vi "get devices and variables.vi"(8 "error in (no error)":errorcluster, 11 "Device":string) -> (0 "error out":errorcluster, 1 "devicetype":string, 2 "variable":string[](array[string]), 3 "Device":string[](array[string]))   [LabVIEW 2013]
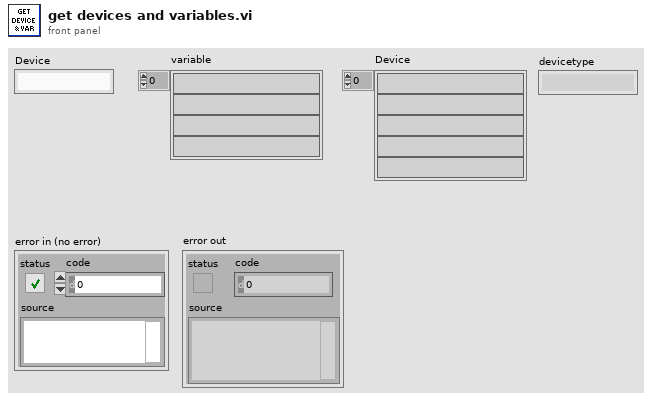
[diagram p1: front panel]
types:
  T1 = typedef "mysql_authentication.ctl" = cluster{"User":string, "Password":string, "Database":string}
  T2 = cluster{"Port":u16, "IP Address":string, "Authentication":T1}
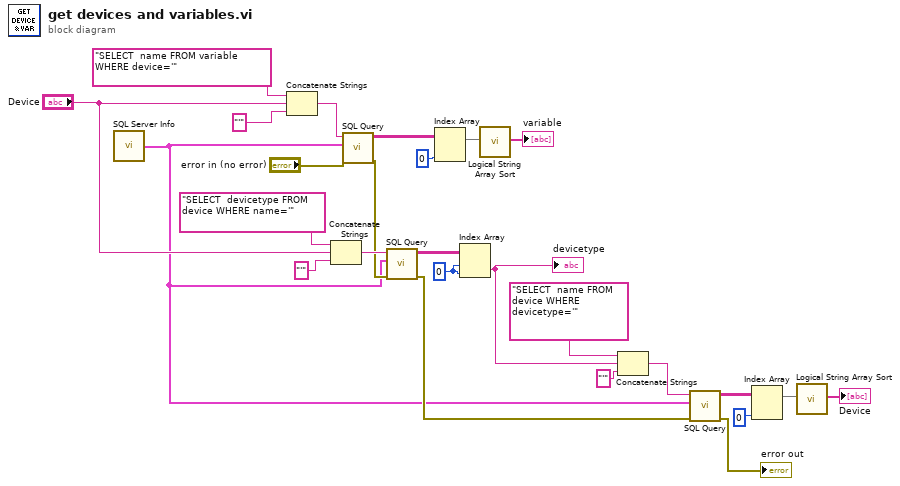
[diagram p0: block diagram]
diagram:
  w7 = 0 ("disabled index (col)")
  n1 = call "SQL Server Info.vi"() -> ("SQL Server Info"=w1:T2)
  n2 = Concatenate Strings("SELECT  name FROM variable WHERE device='" ("Query"), "Device", "'" ("string")) -> (w21:string)
  n3 = Concatenate Strings("SELECT  devicetype FROM device WHERE name='" ("Query"), "Device", "'" ("string")) -> (w8:string)
  n4 = call "SQL Query.vi"("error in (no error)"="error in (no error)", "SQL Server Info"=w1, "Query"=w21) -> ("error out"=w4:errorcluster, "data"=w26:string[][])  [unwired: 7 in]
  n5 = call "SQL Query.vi"("error in (no error)"=w4, "SQL Server Info"=w1, "Query"=w8) -> ("error out"=w3:errorcluster, "data"=w11:string[][])  [unwired: 7 in]
  n6 = Index Array(array=w26, index (col)=0 ("disabled index (col)")) -> (element=w24:string[])  [unwired: 1 in]
  n7 = Index Array(array=w11, index (row)=w7, index (col)=w7) -> (element=w5:string)
  "devicetype" <- w5
  n8 = call "Logical String Array Sort.vi"("Unsorted List"=w24) -> ("Sorted List"=→"variable":string[])  [unwired: 18 in]
  n9 = Concatenate Strings("SELECT  name FROM device WHERE devicetype='" ("Query"), w5, "'" ("string")) -> (w14:string)
  n10 = call "SQL Query.vi"("error in (no error)"=w3, "SQL Server Info"=w1, "Query"=w14) -> ("error out"=→"error out":errorcluster, "data"=w19:string[][])  [unwired: 7 in]
  n11 = Index Array(array=w19, index (col)=0 ("disabled index (col)")) -> (element=w17:string[])  [unwired: 1 in]
  n12 = call "Logical String Array Sort.vi"("Unsorted List"=w17) -> ("Sorted List"=→"Device":string[])  [unwired: 18 in]
